vi "testing perform search.vi"(8 "error in (no error)":errorcluster, 9 "TestSeqId (\"\")":string, 10 "Action (\"Search\")":string="Search", 11 "Connection Refnum":T2) -> (0 "error out":errorcluster, 1 "Matching Results":i32, 2 "Results":T1[](array[typedef]), 3 "Connection Refnum":T2)   [LabVIEW 2011]
uses:
  Summitek EXT/ODBC/SQL Controls/Connection Refnum.ctl
  server/database/Sequences/Sequence Record.ctl
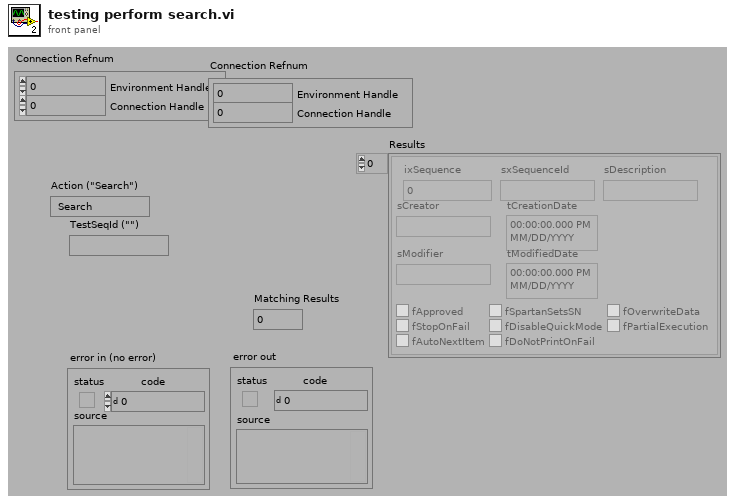
[diagram p1: front panel]
types:
  T1 = typedef "Sequence Record.ctl" = cluster{"ixSequence":i32, "sxSequenceId":string, "sDescription":string, "sCreator":string, "tCreationDate":timestamp, "sModifier":string, "tModifiedDate":timestamp, "fApproved":bool, "fSpartanSetsSN":bool, "fOverwriteData":bool, "fStopOnFail":bool, "fDisableQuickMode":bool, "fPartialExecution":bool, "fAutoNextItem":bool, "fDoNotPrintOnFail":bool}
  T2 = typedef "Connection Refnum.ctl" = cluster{"Environment Handle":i32, "Connection Handle":i32}
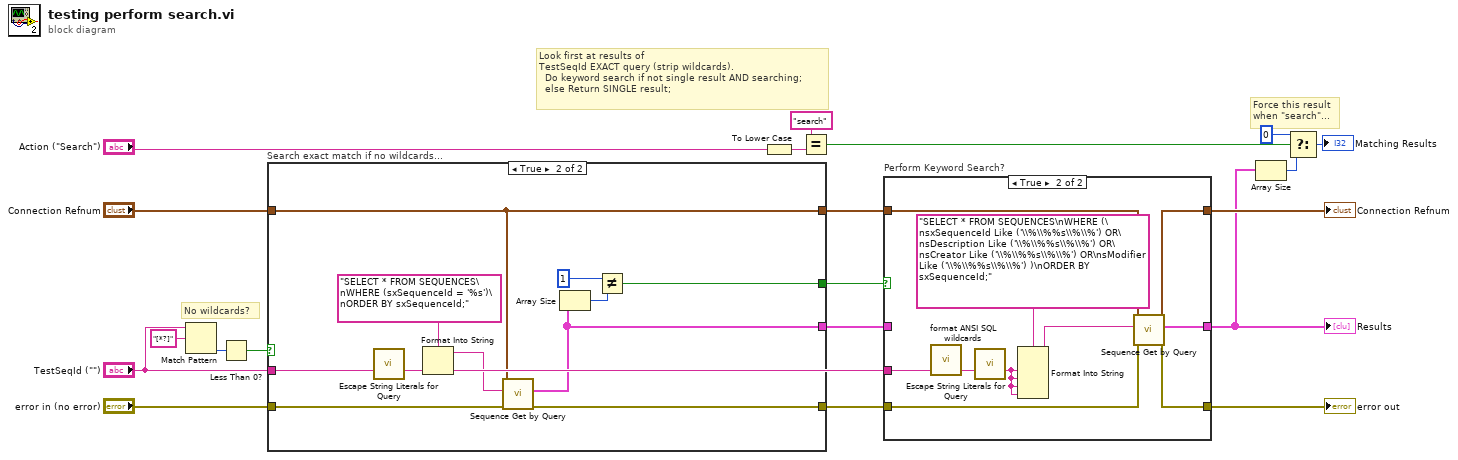
[diagram p0: block diagram]
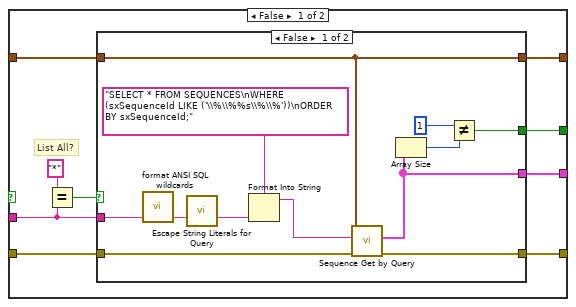
[diagram p2: hidden frame]
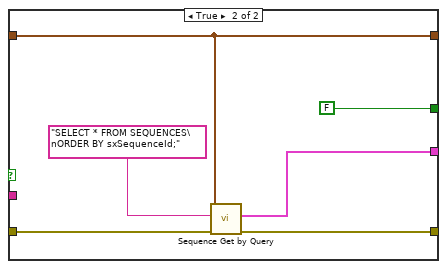
[diagram p3: hidden frame]
diagram:
  # "No wildcards?"
  # "Force this result\nwhen \"search\"..."
  # "Look first at results of\nTestSeqId EXACT query (strip wildcards).\n  Do keyword search if not single result AND searching;\n  else Return SINGLE result;"
  n1 = Match Pattern(string="TestSeqId (\"\")", regular expression="[*?]") -> (offset past match=w11:i32)  [unwired: 4 out]
  n2 = Less Than 0?(x=w11) -> (x < 0?=w9:bool)
  n3 = case "Search exact match if no wildcards..." shown="True" w9 {
    tunnel: "error in (no error)" -> [w27 w51]
    tunnel: [w26 w50] -> w6
    tunnel: "Connection Refnum" -> [w25 w53]
    tunnel: [w23 w53] -> w7
    tunnel: [w29 w55] -> w1
    tunnel: [w24 w52] -> w5
    tunnel: "TestSeqId (\"\")" -> [w22 w54]
    frame False {
      # "List All?"
      n4 = Equal?(x="*" ("regular expression"), y=w22) -> (x = y?=w28:bool)
      n5 = case shown="False" w28 {
        tunnel: [w36 FALSE] -> w29
        tunnel: w27 -> [w34 w45]
        tunnel: [w33 w44] -> w26
        tunnel: w25 -> [w31 w43]
        tunnel: [w30 w42] -> w24
        tunnel: [w31 w43] -> w23
        tunnel: w22 -> [w37 _]
        frame False {
          n6 = call "format ANSI SQL wildcards.vi"("String"=w37) -> ("ANSI SQL Wildcard String"=w41:string)  [unwired: 4 out]
          n7 = call "Escape String Literals for Query.vi"("String"=w41) -> ("escaped String"=w40:string)  [unwired: 1 in, 13 out]
          n8 = Format Into String(format string="SELECT * FROM SEQUENCES\nWHERE (sxSequenceId LIKE ('\\%\\%%s\\%\\%'))\nORDER BY sxSequenceId;" ("User Query"), w40) -> (resulting string=w32:string)  [unwired: 2 in, 1 out]
          n9 = call "Sequence Get by Query.vi"("error in (no error)"=w34, "Sequence Query (\"\")"=w32, "Connection Refnum"=w31) -> ("error out"=w33:errorcluster, "Records"=w30:T1[])  [unwired: 7 out]
          n10 = Array Size(array=w30) -> (size(s)=w38:i32)
          n11 = Not Equal?(x=1, y=w38) -> (x != y?=w36:bool)
        }
        frame True {
          n12 = call "Sequence Get by Query.vi"("error in (no error)"=w45, "Sequence Query (\"\")"="SELECT * FROM SEQUENCES\nORDER BY sxSequenceId;" ("User Query"), "Connection Refnum"=w43) -> ("error out"=w44:errorcluster, "Records"=w42:T1[])  [unwired: 7 out]
        }
      }
    }
    frame True {
      n13 = call "Escape String Literals for Query.vi"("String"=w54) -> ("escaped String"=w58:string)  [unwired: 1 in, 13 out]
      n14 = Format Into String(format string="SELECT * FROM SEQUENCES\nWHERE (sxSequenceId = '%s')\nORDER BY sxSequenceId;" ("User Query"), w58) -> (resulting string=w49:string)  [unwired: 2 in, 1 out]
      n15 = call "Sequence Get by Query.vi"("error in (no error)"=w51, "Sequence Query (\"\")"=w49, "Connection Refnum"=w53) -> ("error out"=w50:errorcluster, "Records"=w52:T1[])  [unwired: 7 out]
      n16 = Array Size(array=w52) -> (size(s)=w56:i32)
      n17 = Not Equal?(x=1, y=w56) -> (x != y?=w55:bool)
    }
  }
  n18 = To Lower Case(string="Action (\"Search\")") -> (all lower case string=w3:string)
  n19 = Equal?(x="search", y=w3) -> (x = y?=w16:bool)
  n20 = case "Perform Keyword Search?" shown="True" w1 {
    tunnel: w7 -> [w60 w71]
    tunnel: w6 -> [w59 w69]
    tunnel: [w60 w70] -> w19
    tunnel: "TestSeqId (\"\")" -> [_ w63]
    tunnel: w5 -> [w61 _]
    tunnel: [w61 w67] -> w17
    tunnel: [w59 w66] -> w18
    frame False {
    }
    frame True {
      n21 = call "format ANSI SQL wildcards.vi"("String"=w63) -> ("ANSI SQL Wildcard String"=w64:string)  [unwired: 4 out]
      n22 = call "Escape String Literals for Query.vi"("String"=w64) -> ("escaped String"=w62:string)  [unwired: 1 in, 13 out]
      n23 = Format Into String(format string="SELECT * FROM SEQUENCES\nWHERE (\nsxSequenceId Like ('\\%\\%%s\\%\\%') OR\nsDescription Like ('\\%\\%%s\\%\\%') OR\nsCreator Like ('\\%\\%%s\\%\\%') OR\nsModifier Like ('\\%\\%%s\\%\\%') )\nORDER BY sxSequenceId;" ("User Query"), w62, w62, w62, w62) -> (resulting string=w65:string)  [unwired: 2 in, 1 out]
      n24 = call "Sequence Get by Query.vi"("error in (no error)"=w69, "Sequence Query (\"\")"=w65, "Connection Refnum"=w71) -> ("error out"=w66:errorcluster, "Records"=w67:T1[], "Connection Refnum"=w70:T2)  [unwired: 6 out]
    }
  }
  "error out" <- w18
  "Connection Refnum" <- w19
  "Results" <- w17
  n25 = Array Size(array=w17) -> (size(s)=w15:i32)
  n26 = Select(t=0, s=w16, f=w15) -> (s? t:f=→"Matching Results":i32)
